vi "Curing inf.vi"(7 "write\\read（read)":enum16{"read", "write"}(ring), 9 "value in":dbl caption="值", 10 "key":string caption="键", 11 "path in":path) -> (2 "value out":dbl caption="值", 3 "path out":path)   [LabVIEW 2014]
uses:
  <vilib>/Utility/config.llb/Read Key (Double).vi
  <vilib>/Utility/config.llb/Write Key (Double).vi
  <vilib>/Utility/config.llb/NI_LVConfig.lvlib
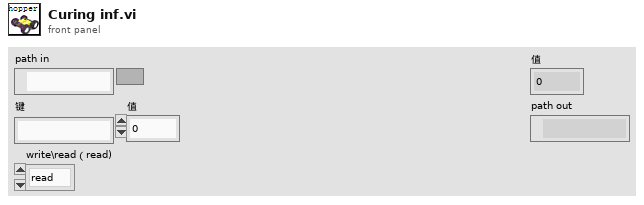
[diagram p1: front panel]
types:
  T1 = typedef "NI_LVConfig.lvlib/Config Data RefNum.ctl" = refnum<k1>
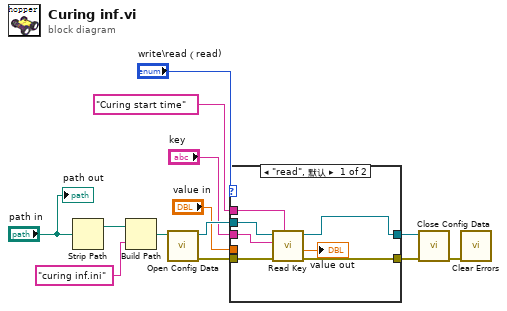
[diagram p0: block diagram]
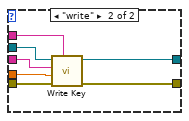
[diagram p2: hidden frame]
diagram:
  n1 = Strip Path(path="path in") -> (stripped path=w13:path)  [unwired: 1 out]
  n2 = Build Path(base path=w13, name or relative path="curing inf.ini" ("名称或相对路径")) -> (appended path=w11:path)
  n3 = call <vilib>:"Open Config Data.vi"("configuration file path"=w11) -> ("error out"=w10:errorcluster, "refnum"=w9:T1)  [unwired: 8 in, 1 out]
  n4 = case shown="\"read\", 默认" "write\\read（read)" {
    tunnel: w10 -> [w18 w27]
    tunnel: w9 -> [w19 w26]
    tunnel: "Curing start time" ("section") -> [w16 w25]
    tunnel: [w17 w24] -> w7
    tunnel: [w20 w23] -> w6
    tunnel: "key" -> [w15 w22]
    tunnel: "value in" -> [_ w21]
    frame "read", Default {
      n5 = call-poly <vilib>:"Read Key.vi"("section"=w16, "error in (no error)"=w18, "key"=w15, "refnum"=w19) -> ("error out"=w20:errorcluster, "value"=→"value out":dbl, "refnum out"=w17:T1)  [unwired: 4 in, 1 out]
    }
    frame "write" {
      n6 = call-poly <vilib>:"Write Key.vi"("section"=w25, "error in (no error)"=w27, "value"=w21, "key"=w22, "refnum"=w26) -> ("error out"=w23:errorcluster, "refnum out"=w24:T1)  [unwired: 4 in, 1 out]
    }
  }
  n7 = call <vilib>:"Close Config Data.vi"("error in (no error)"=w6, "refnum"=w7) -> ("error out"=w3:errorcluster)  [unwired: 8 in, 1 out]
  n8 = call <vilib>:"Clear Errors.vi"("error in (no error)"=w3) -> ()  [unwired: 5 in, 2 out]
  "path out" <- "path in"
